vi "ConvertMsgs.vi"(11 "Message Type":string) -> (3 "result string":string)   [LabVIEW 2022 SP3]
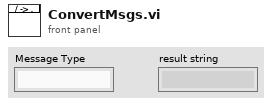
[diagram p1: front panel]
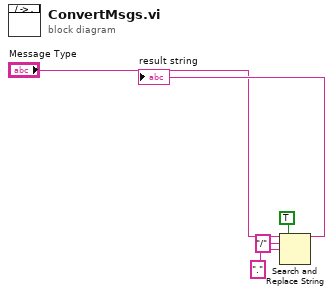
[diagram p0: block diagram]
diagram:
  n1 = Search and Replace String(replace all?=TRUE ("replace all? (F)"), input string="Message Type", search string="/", replace string="." ("search string")) -> (result string=→"result string":string)  [unwired: 4 in, 3 out]
